vi "Element Type.vi"(11 "SimpleChart in":refnum<class "SimpleChart.lvclass">) -> (2 "Element Type":string)   [LabVIEW 2020, in "VolatusGUIElements.lvlib" / "SimpleChart.lvclass"]
uses:
  SimpleChart.lvclass
  SimpleChart.lvclass/SimpleChart.ctl
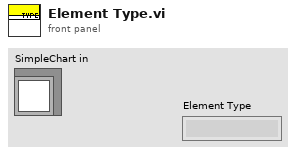
[diagram p1: front panel]
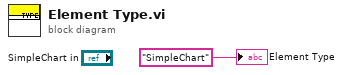
[diagram p0: block diagram]
diagram:
  "Element Type" <- "SimpleChart" ("Element Type")
